vi "PH_PP_CurrentMeas_Status.vi"(0 "connection ID in":refnum<k5>, 2 "NI6071E DAQ Server":string="dveert01.gsi.de", 3 "Port":u16, 5 "error in (no error)":errorcluster) -> (14 "connection ID out":refnum<k5>, 15 "Error unpacking Data?":bool, 16 "Connection not established":bool, 17 "Receveived Data Sets":T1[](array[typedef]), 19 "error out":errorcluster)   [LabVIEW 2014, in "PH_PP_CurrentMeas.lvlib"]
uses:
  PH_PP_CurrentMeas.lvlib
  PH_PP_CurrentMeas.Command.ctl
  PH_PP_CurrentMeas.CommandCluster.ctl
panel:
  in  "Dummy":T1
  in  "Command":T2=enum."CloseConnection"
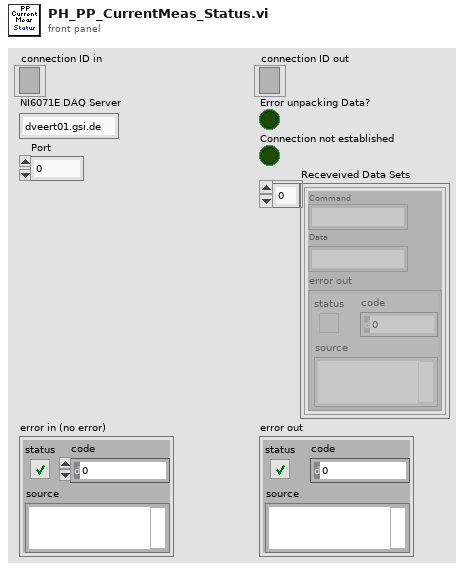
[diagram p1: front panel]
types:
  T1 = typedef "PH_PP_CurrentMeas.lvlib/PH_PP_CurrentMeas.CommandCluster.ctl" = cluster{"Command":string, "Data":string, "error out":errorcluster}
  T2 = typedef "PH_PP_CurrentMeas.lvlib/PH_PP_CurrentMeas.Command.ctl" = enum16{"StartDAQ", "StopDAQ", "GetDAQStatus", "CloseConnection"}
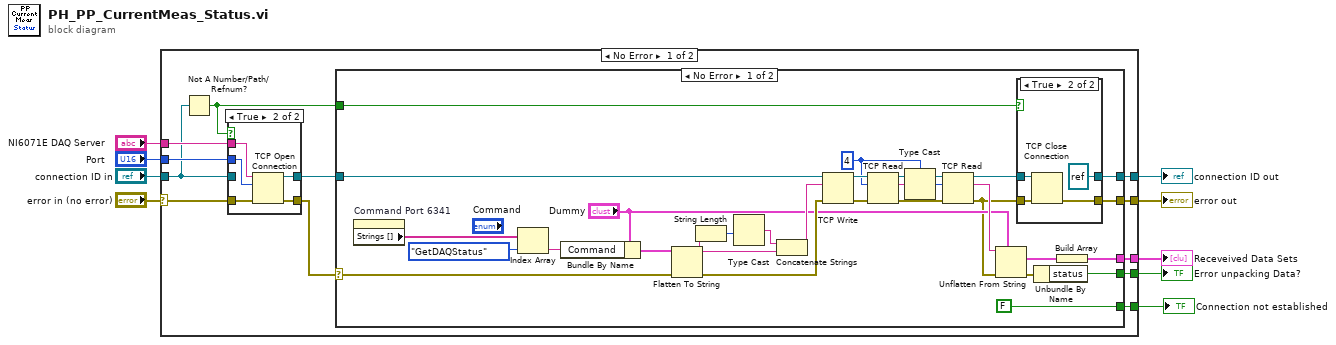
[diagram p0: block diagram]
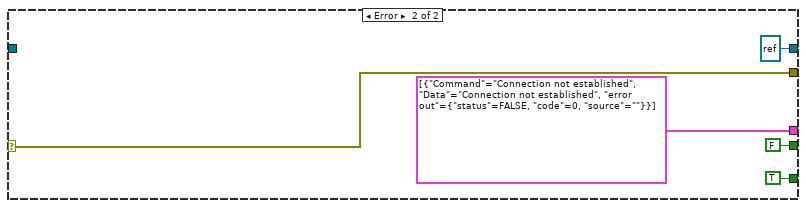
[diagram p3: hidden frame]
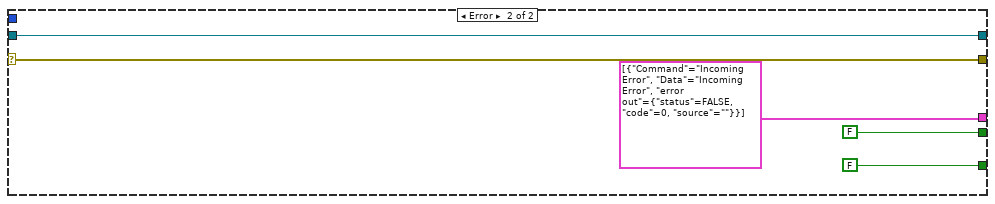
[diagram p5: hidden frame]
diagram:
  n1 = case shown="No Error" "error in (no error)" {
    selector: "error in (no error)" -> [w12 w74]
    tunnel: [w21 w73] -> w9
    tunnel: [w20 w74] -> w8
    tunnel: [w19 T1[] [{"Command"="Incoming Error", "Data"="Incoming Error", "error out"={"status"=FALSE, "code"=0, "source"=""}}]] -> w7
    tunnel: [w18 FALSE ("status")] -> w6
    tunnel: "Port" -> [w16 _]
    tunnel: "NI6071E DAQ Server" -> [w15 _]
    tunnel: "connection ID in" -> [w14 w73]
    tunnel: [w10 FALSE] -> w1
    frame No Error {
      n2 = Not A Number/Path/Refnum?(number/path/refnum=w14) -> (NaN/Path/Refnum?=w17:bool)
      n3 = case shown="True" w17 {
        tunnel: w14 -> [w63 _]
        tunnel: w12 -> [w64 w69]
        tunnel: [w64 w68] -> w11
        tunnel: w16 -> [_ w67]
        tunnel: w15 -> [_ w66]
        tunnel: [w63 w65] -> w13
        frame False {
        }
        frame True {
          n4 = TCP Open Connection(address=w66, remote port or service name=w67, error in (no error)=w69) -> (connection ID=w65:refnum<k5>, error out=w68:errorcluster)  [unwired: 2 in]
        }
      }
      n5 = case shown="No Error" w11 {
        selector: w11 -> [w23 w62]
        tunnel: [w51 refnum<k5> refnum ("connection ID")] -> w21
        tunnel: [w50 w62] -> w20
        tunnel: [w49 T1[] [{"Command"="Connection not established", "Data"="Connection not established", "error out"={"status"=FALSE, "code"=0, "source"=""}}]] -> w19
        tunnel: [w48 FALSE ("status")] -> w18
        tunnel: w17 -> [w25 _]
        tunnel: w13 -> [w24 _]
        tunnel: [FALSE TRUE] -> w10
        frame No Error {
          w30 = 4 ("bytes to read")
          n6 = property on="Command Port 6341" class="Enum (strict)"() -> ("Strings []"=w31:string[])  [unwired: 2 in, 2 out]
          n7 = Index Array(array=w31, index=PH_PP_CurrentMeas.Command."GetDAQStatus" ("Command")) -> (element=w47:string)
          n8 = Bundle By Name(cluster="Dummy", "Command"=w47) -> (w42:T1)
          n9 = Flatten To String(anything=w42, error in (no error)=w23) -> (data string=w44:string, error out=w41:errorcluster)  [unwired: 2 in, 1 out]
          n10 = String Length(string=w44) -> (length=w45:i32)
          n11 = Type Cast(x=w45) -> (*(type *) &x=w46:string)  [unwired: 1 in]
          n12 = Concatenate Strings(w46, w44) -> (w43:string)
          n13 = TCP Write(connection ID=w24, data in=w43, error in (no error)=w41) -> (connection ID out=w34:refnum<k5>, error out=w35:errorcluster)  [unwired: 1 in, 1 out]
          n14 = TCP Read(connection ID=w34, bytes to read=w30, error in (no error)=w35) -> (connection ID out=w38:refnum<k5>, data out=w36:string, error out=w39:errorcluster)  [unwired: 2 in]
          n15 = Type Cast(type=w30, x=w36) -> (*(type *) &x=w37:i32)
          n16 = TCP Read(connection ID=w38, bytes to read=w37, error in (no error)=w39) -> (connection ID out=w26:refnum<k5>, data out=w40:string, error out=w27:errorcluster)  [unwired: 2 in]
          n17 = Unflatten From String(type="Dummy", binary string=w40, error in (no error)=w27) -> (value=w29:T1, error out=w28:errorcluster)  [unwired: 2 in, 1 out]
          n18 = case shown="True" w25 {
            tunnel: [w53 refnum<k5> refnum ("connection ID")] -> w51
            tunnel: [w52 w57] -> w50
            tunnel: w27 -> [w52 w56]
            tunnel: w26 -> [w53 w55]
            frame False {
            }
            frame True {
              n19 = TCP Close Connection(connection ID=w55, error in (no error)=w56) -> (error out=w57:errorcluster)  [unwired: 1 in, 1 out]
            }
          }
          n20 = Unbundle By Name(w28) -> ("status"=w48:bool)
          n21 = Build Array(w29) -> (w49:T1[])
        }
        frame Error {
        }
      }
    }
    frame Error {
    }
  }
  "connection ID out" <- w9
  "error out" <- w8
  "Receveived Data Sets" <- w7
  "Error unpacking Data?" <- w6
  "Connection not established" <- w1
